vi "KRH Solenoid.vi"(8 "Input":bool, 9 "Time On Delay":i32, 10 "Pulse Width (ms)":i32, 11 "Ref 0":string) -> (2 "Status":bool)   [LabVIEW 2015]
uses:
  <vilib>/Rock Robotics/WPI/Solenoid/WPI_SolenoidSetEnum.vi
panel:
  in  "String 4":string
  in  "String 3":string
  in  "String 2":string
  in  "String":string
  in  "Ref 2":string
  in  "Ref 1":string
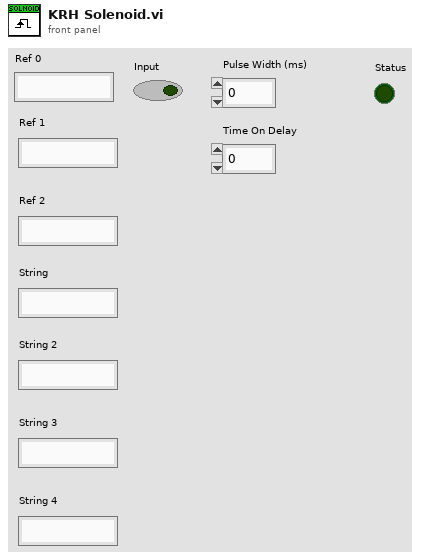
[diagram p1: front panel]
types:
  T1 = typedef "WPI_SolenoidDevRef.ctl" = cluster{"DevStatus":errorcluster, "Pneumatics Control Module":u8, "Forward Solenoid Channel":T2, "Reverse Solenoid Channel":T2}
  T2 = typedef "WPI_SolenoidChannel.ctl" = enum8{"Solenoid 0", "Solenoid 1", "Solenoid 2", "Solenoid 3", "Solenoid 4", "Solenoid 5", "Solenoid 6", "Solenoid 7", "Invalid"}
  T3 = typedef "WPI_SolenoidValue.ctl" = enum16{"Off", "On", "Forward", "Reverse"}
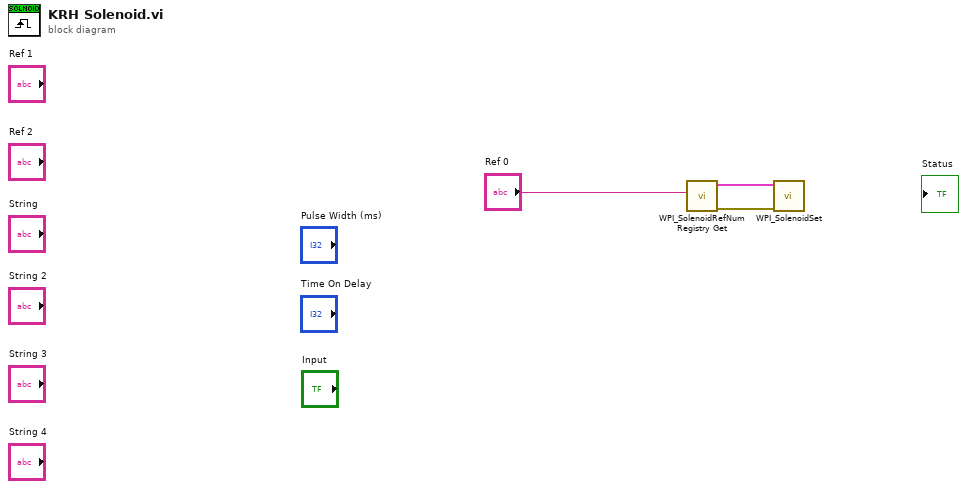
[diagram p0: block diagram]
diagram:
  n1 = call <vilib>:"WPI_SolenoidRefNum Registry Get.vi"("refnum name"="Ref 0") -> ("error out"=w1:errorcluster, "SolenoidDevRef"=w4:T1)  [unwired: 9 in]
  n2 = call-poly <vilib>:"WPI_SolenoidSet.vi"("error in (no error)"=w1, "SolenoidDevRef"=w4) -> ("Value"=w2:T3)  [unwired: 7 in, 2 out]
